vi "Get-Set Properties from Cluster (logInfo).vi"() -> ()   [LabVIEW 2020]
uses:
  Shared/logFileInfo_types.ctl
  Scripting/AIM ARINC 664 Scripting.lvlib
panel:
  out "x = y?":T1
  out "read":T2
  in  "log file info":T2={"Log Directory"="/c/ni-rt/NIVeriStand/Logs", "Base Name"="AIM664log", "Timestamp"=FALSE, "Enabled"=FALSE}
  # "Set UNIT_TEST \nconditional disable symbol\nto T to test"
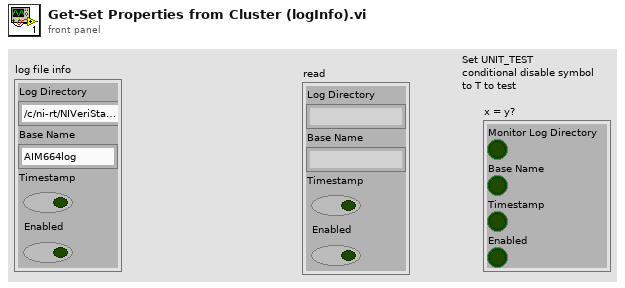
[diagram p1: front panel]
types:
  T1 = cluster{"Monitor Log Directory":bool, "Base Name":bool, "Timestamp":bool, "Enabled":bool}
  T2 = typedef "logFileInfo_types.ctl" = cluster{"Log Directory":string, "Base Name":string, "Timestamp":bool, "Enabled":bool}
  T3 = cluster{"Log Directory":bool, "Base Name":bool, "Timestamp":bool, "Enabled":bool}
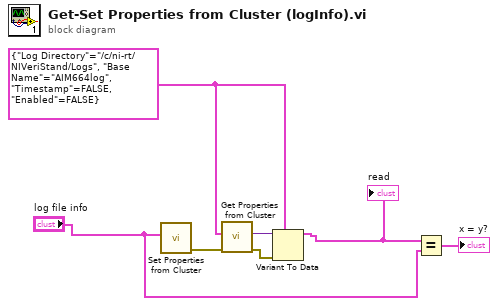
[diagram p0: block diagram]
diagram:
  w5 = T2 {"Log Directory"="/c/ni-rt/NIVeriStand/Logs", "Base Name"="AIM664log", "Timestamp"=FALSE, "Enabled"=FALSE} ("log file info")
  n1 = call "Set Properties from Cluster.vi"("Variant Cluster"="log file info") -> ("error out"=w4:errorcluster)  [unwired: 9 in, 1 out]
  n2 = call "Get Properties from Cluster.vi"("error in"=w4, "Variant Cluster"=w5) -> ("error out"=w6:errorcluster, "data"=w7:variant)  [unwired: 6 in, 2 out]
  n3 = Variant To Data(error in=w6, type=w5, Variant=w7) -> (data=w2:T2)  [unwired: 1 out]
  "read" <- w2
  n4 = Equal?(x=w2, y="log file info") -> (x = y?=→"x = y?":T3)
